vi "Operation.vi"(8 "Error In":errorcluster, 11 "Divide In":refnum<class "Divide.lvclass">) -> (0 "Error Out":errorcluster, 2 "C":dbl, 3 "Divide Out":refnum<class "Divide.lvclass">)   [LabVIEW 2023, in "Divide.lvclass"]
doc: "The VI performs the division operation for two numbers and displays the output."
uses:
  Divide.lvclass
  Divide.lvclass/Divide.ctl
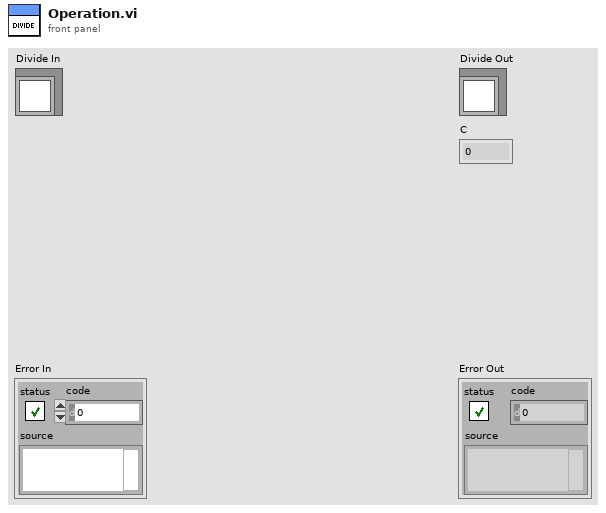
[diagram p1: front panel]
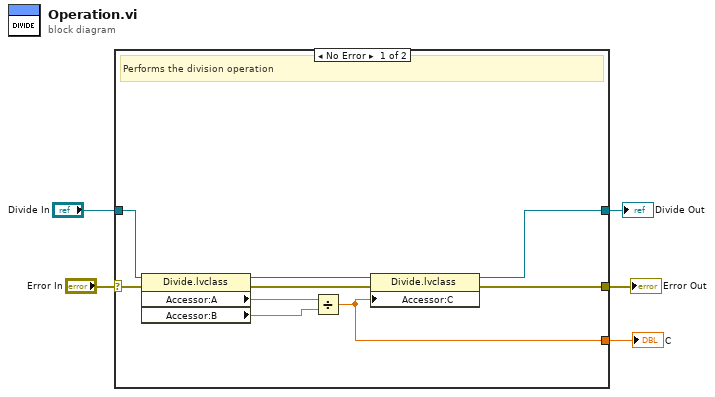
[diagram p0: block diagram]
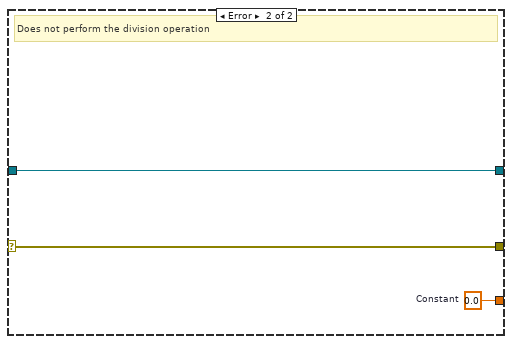
[diagram p2: hidden frame]
diagram:
  n1 = case shown="No Error" "Error In" {
    selector: "Error In" -> [w14 w17]
    tunnel: [w9 w17] -> w4
    tunnel: [w6 w16] -> w2
    tunnel: "Divide In" -> [w12 w16]
    tunnel: [w7 w15] -> w1
    frame No Error {
      # "Performs the division operation"
      n2 = property class="Divide.lvclass"(reference=w12, error in=w14) -> (reference out=w8:refnum<class "Divide.lvclass">, error out=w13:errorcluster, "Accessor:A"=w11:dbl, "Accessor:B"=w10:dbl)
      n3 = Divide(x=w11, y=w10) -> (x/y=w7:dbl)
      n4 = property class="Divide.lvclass"(reference=w8, error in=w13, "Accessor:C"=w7) -> (reference out=w6:refnum<class "Divide.lvclass">, error out=w9:errorcluster)
    }
    frame Error {
      w15 = 0.0  # Constant
      # "Does not perform the division operation"
    }
  }
  "Error Out" <- w4
  "Divide Out" <- w2
  "C" <- w1
